vi "Pump_Status.vi"(8 "error in (no error)":errorcluster, 10 "Default State":T1, 11 "reference":refnum<visa-resource-name>) -> (2 "Next State":T1=enum."Wait for Event")   [LabVIEW 2024]
uses:
  controls/State.ctl
panel:
  out "error out":errorcluster
  out "read buffer":string
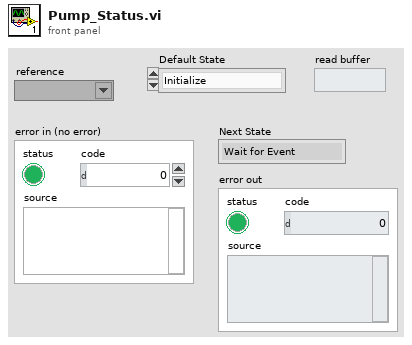
[diagram p1: front panel]
types:
  T1 = typedef "State.ctl" = enum16{"Initialize", "Wait for Event", "Position", "Valve Signal", "Extra Flush", "Valve Cycle", "Valve Open", "Valve Close", "Pump Command", "Pump Cycle", "Empty System", "Start System", "Connect Systems", "Start Image Capture", "Stop Image Capture", "Calibration Pictures", "StatusRequest", "RequestBarcodes", "SendBarcode", "ReturnHome", "ReInit. F3", "Clear F3 Error", "CursorIdle", "Exit"}
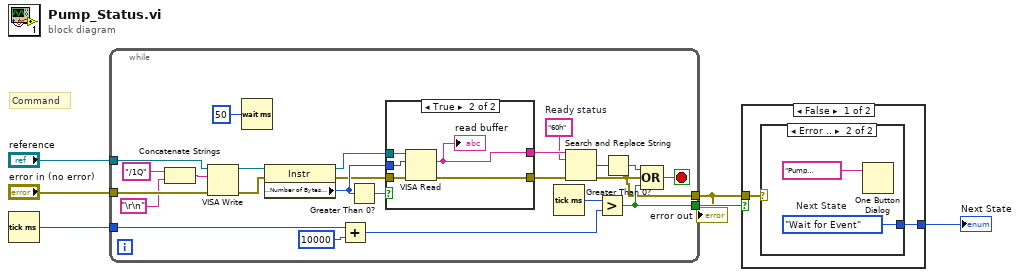
[diagram p0: block diagram]
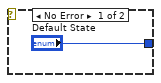
[diagram p2: hidden frame]
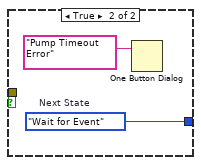
[diagram p3: hidden frame]
diagram:
  # "Command"
  n1 = Tick Count (ms)() -> (millisecond timer value=w6:u32)
  n2 = while {
    tunnel: w6 -> [w17]
    tunnel: "error in (no error)" -> [w12]
    tunnel: [w11] -> w4
    tunnel: [w10] -> w2
    tunnel: "reference" -> [w9]
    stop <- w21 stop-if-true
    w24 = "60h"  # Ready status
    n3 = Concatenate Strings("/1Q" ("write buffer"), "\r\n") -> (w8:string)
    n4 = VISA Write(VISA resource name=w9, write buffer=w8, error in (no error)=w12) -> (VISA resource name out=w14:refnum<visa-resource-name>, error out=w13:errorcluster)  [unwired: 1 out]
    n5 = Wait (ms)(milliseconds to wait=u32 50) -> ()  [unwired: 1 out]
    n6 = property class="Instr"(reference=w14, error in=w13) -> (reference out=w26:refnum<visa-resource-name>, error out=w27:errorcluster, "Serial Settings:Number of Bytes at Serial Port"=w29:u32)
    n7 = Add(x=w17, y=u32 10000) -> (x+y=w18:u32)
    n8 = Greater Than 0?(x=w29) -> (x > 0?=w28:bool)
    n9 = case shown="True" w28 {
      tunnel: w26 -> [_ w36]
      tunnel: w27 -> [w31 w35]
      tunnel: [w31 w34] -> w22
      tunnel: w29 -> [_ w33]
      tunnel: [_ w32] -> w25
      frame False {
      }
      frame True {
        n10 = VISA Read(VISA resource name=w36, byte count=w33, error in (no error)=w35) -> (read buffer=w32:string, error out=w34:errorcluster)  [unwired: 2 out]
        "read buffer" <- w32
      }
    }
    n11 = Tick Count (ms)() -> (millisecond timer value=w19:u32)
    n12 = Search and Replace String(input string=w25, search string=w24, error in=w22) -> (number of replacements=w23:i32, error out=w10:errorcluster)  [unwired: 5 in, 2 out]
    n13 = Greater?(x=w19, y=w18) -> (0:w11:bool)
    n14 = Greater Than 0?(x=w23) -> (x > 0?=w20:bool)
    n15 = Compound Arithmetic op=OR(w20, w10, w11) -> (w21:bool)
  }
  "error out" <- w2
  n16 = case shown="False" w4 {
    tunnel: [w37 w43] -> w3
    tunnel: w2 -> [w38 _]
    frame False {
      n17 = case shown="Error .." w38 {
        tunnel: ["Default State" w41] -> w37
        frame No Error {
        }
        frame Error {
          w41 = State."Wait for Event"  # Next State
          n18 = One Button Dialog(message="Pump Connection Error") -> ()  [unwired: 1 in, 1 out]
        }
      }
    }
    frame True {
      w43 = State."Wait for Event"  # Next State
      n19 = One Button Dialog(message="Pump Timeout Error") -> ()  [unwired: 1 in, 1 out]
    }
  }
  "Next State" <- w3
